vi "Ascenseur_Controller.vi"() -> ()   [LabVIEW 2019]
uses:
  <vilib>/myRIO/Instrument Drivers/Onboard IO/DIO/DIO.lvlib
  Commande 2.ctl
  <vilib>/myRIO/Common/Instrument Driver Framework/myRIO v1.0/DIO/typedefs/DIO Channels Enum.ctl
  <vilib>/myRIO/Common/Instrument Driver Framework/myRIO v1.0/DIO/typedefs/DIO Channels List.ctl
  <vilib>/myRIO/Common/Instrument Driver Framework/Utilities/typedefs/Generic FPGA Reference.ctl
  <vilib>/myRIO/Common/Instrument Driver Framework/Utilities/typedefs/myRIO v1.0 Reference.ctl
  <vilib>/myRIO/Common/Instrument Driver Framework/Utilities/typedefs/Hardware Version Enum.ctl
  <vilib>/myRIO/Common/Instrument Driver Framework/Utilities/typedefs/myRIO Generic Hardware Reference.ctl
  <vilib>/myRIO/Instrument Drivers/Onboard IO/DIO/typedefs/DIO Reference.ctl
  <vilib>/myRIO/Instrument Drivers/Onboard IO/DIO/vis/myRIO DIO Open.xnode
  <vilib>/myRIO/Common/Instrument Driver Framework/myRIO v1.0/DIO/vis/myRIO v1.1 Open DIO.vi
  <vilib>/userDefined/High Color/nirio_resource_hc.ctl
  L298N_Driver/L298N_Ref_Type.ctl
panel:
  in  "Bouton Stop":bool
  out "Var_Etat":T1
  in  "PF_0":bool
  in  "PF_3":bool
  in  "PF_2":bool
  in  "PF_1":bool
  in  "PO_0":bool
  in  "PO_3":bool
  in  "PO_2":bool
  in  "PO_1":bool
  out "Moteur Porte 3":bool
  out "Moteur Porte 2":bool
  out "Moteur Porte 1":bool
  out "Moteur Porte 0":bool
  out "Moteur Cabine":bool
  in  "P0":bool
  in  "P3":bool
  in  "P2":bool
  in  "P1":bool
  in  "Etat_Asc":T1
  in  "Dest_3":bool
  in  "Dest_2":bool
  in  "Dest_1":bool
  in  "Dest_0":bool
  in  "Appel_0":bool
  in  "Appel_3":bool
  in  "Appel_2":bool
  in  "Appel_1":bool
  out "Cluster":T2
  in  "Énum":T3(ring)
  out "Etat":string
  out "Etat Ouvrir Porte 1":bool
  in  "Ouvrir Porte 1":bool
  out "error out 4":errorcluster caption="error out"
  in  "error in (no error) 4":errorcluster caption="error in (no error)"
  in  "Fermer  Porte 1":bool
  out "error out 3":errorcluster caption="error out"
  in  "error in (no error) 3":errorcluster caption="error in (no error)"
  out "error out 2":errorcluster caption="error out"
  in  "error in (no error) 2":errorcluster caption="error in (no error)"
  in  "Cabine Descendre":bool
  out "error out":errorcluster
  in  "error in (no error)":errorcluster
  in  "Cabine Monter":bool
  # "Simulation de présence cabine"
  # "Simulation de portes"
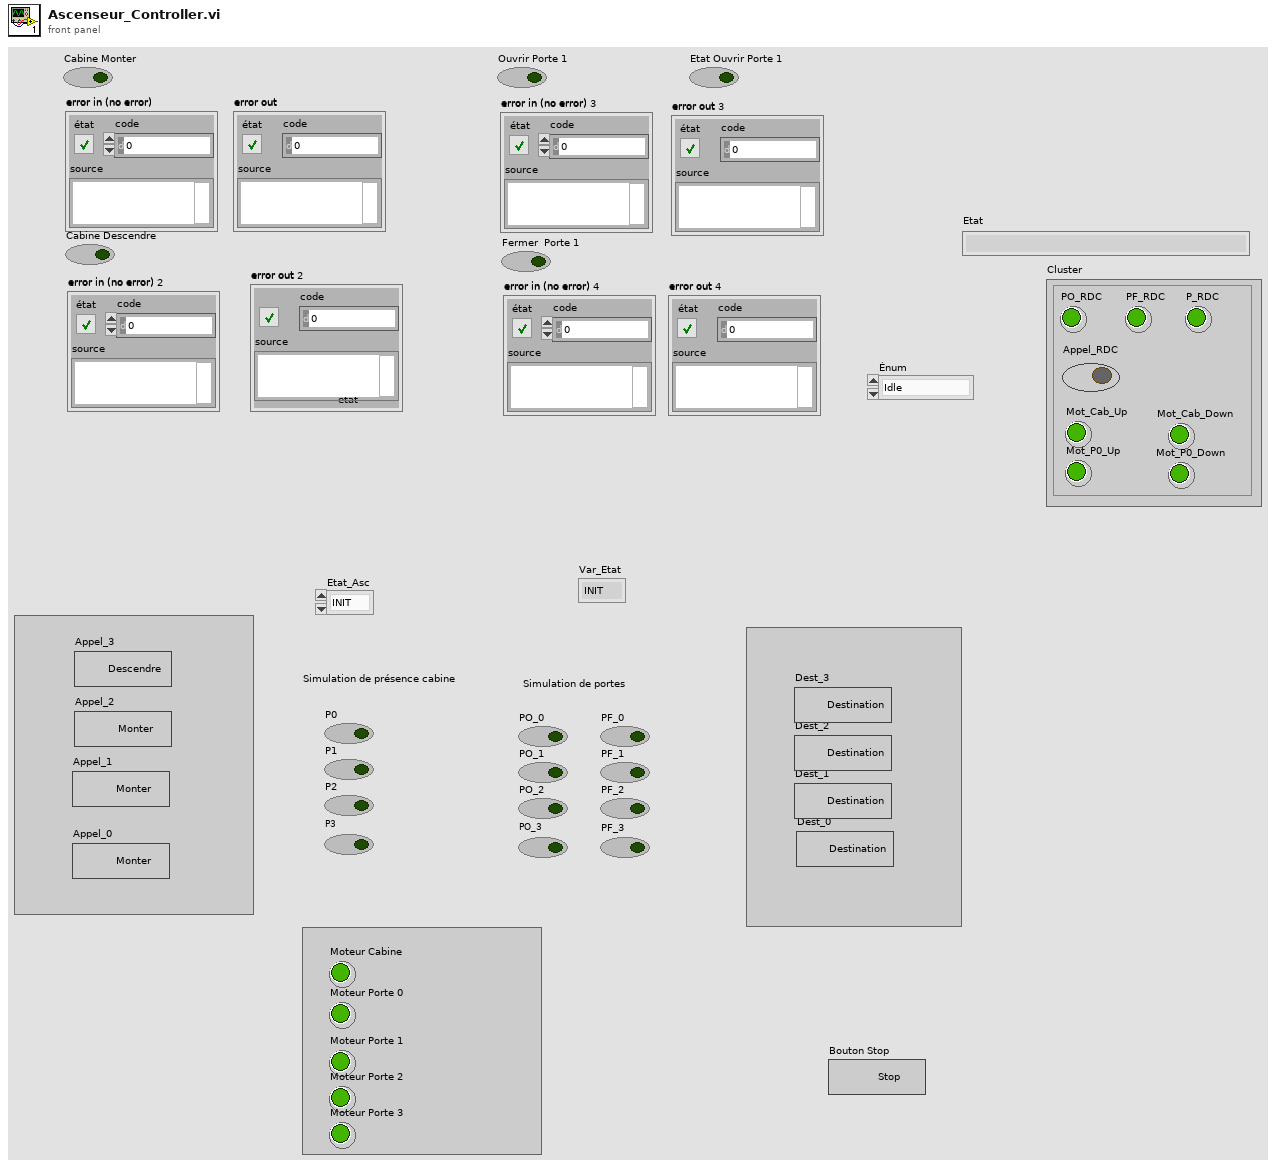
[diagram p1: front panel]
types:
  T1 = typedef "Commande 2.ctl" = enum16{"INIT", "REPOS", "DEPLACEMENT", "OUVERTURE_PORTE", "ATTENTE_TEMPO", "FERMETURE_PORTE", "ARRET_URGENCE"}
  T2 = cluster{"PO_RDC":bool, "PF_RDC":bool, "P_RDC":bool, "Appel_RDC":bool, "Mot_Cab_Up":bool, "Mot_Cab_Down":bool, "Mot_P0_Up":bool, "Mot_P0_Down":bool}
  T3 = enum16{"Idle", "Appel_Etage0", "Descente_Cabine", "Arrivee_Etage0", "Ouverture_Porte", "Attente_Porte", "Fermerture_Porte", "Fin", ""}
  T4 = typedef "L298N_Ref_Type.ctl" = cluster{"DIO_Ref_Montee":T5, "DIO_Ref_Descente":T5}
  T5 = typedef "DIO.lvlib/DIO Reference.ctl" = cluster{"myRIO Reference":T6, "DIO Channels List":T10}
  T6 = typedef "myRIO Generic Hardware Reference.ctl" = cluster{"myRIO Model":T7, "myRIO Hardware Reference":T8}
  T7 = typedef "Hardware Version Enum.ctl" = enum16{"Unknown", "myRIO-1900", "myRIO-1950", "roboRIO", "NI ELVIS RIO CM", "ELVIS III"}
  T8 = typedef "myRIO v1.0 Reference.ctl" = cluster{"Generic FPGA Reference":T9, "Allow multiple opens":bool}
  T9 = typedef "Generic FPGA Reference.ctl" = refnum<k20>
  T10 = typedef "DIO Channels List.ctl" = T11[]
  T11 = typedef "DIO Channels Enum.ctl" = enum16{"Not Connected", "C/DIO0", "C/DIO1", "C/DIO2", "C/DIO3", "C/DIO4", "C/DIO5", "C/DIO6", "C/DIO7", "A/DIO0", "A/DIO1", "A/DIO2", "A/DIO3", "A/DIO4", "A/DIO5", "A/DIO6", "A/DIO7", "A/DIO8", "A/DIO9", "A/DIO10", "A/DIO11", "A/DIO12", "A/DIO13", "A/DIO14", "A/DIO15", "A/DIO16", "A/DIO17", "A/DIO18", "A/DIO19", "B/DIO0", "B/DIO1", "B/DIO2", "B/DIO3", "B/DIO4", "B/DIO5", "B/DIO6", "B/DIO7", "B/DIO8", "B/DIO9", "B/DIO10", "B/DIO11", "B/DIO12", "B/DIO13", "B/DIO14", "B/DIO15", "B/DIO16", "B/DIO17", "B/DIO18", "B/DIO19", "LED0", "LED1", "LED2", "LED3", "Button0", "DIO/DIO0", "DIO/DIO1", "DIO/DIO2", "DIO/DIO3", "DIO/DIO4", "DIO/DIO5", "DIO/DIO6", "DIO/DIO7", "DIO/DIO8", "DIO/DIO9", "SPI/CS0", "SPI/CS1", "SPI/CS2", "SPI/CS3", "LED RADIO (Green)", "LED RADIO (Red)", "LED COMM (Green)", "LED COMM (Red)", "LED MODE (Green)", "LED MODE (Red)"}
  T12 = typedef "nirio_resource_hc.ctl" = tag
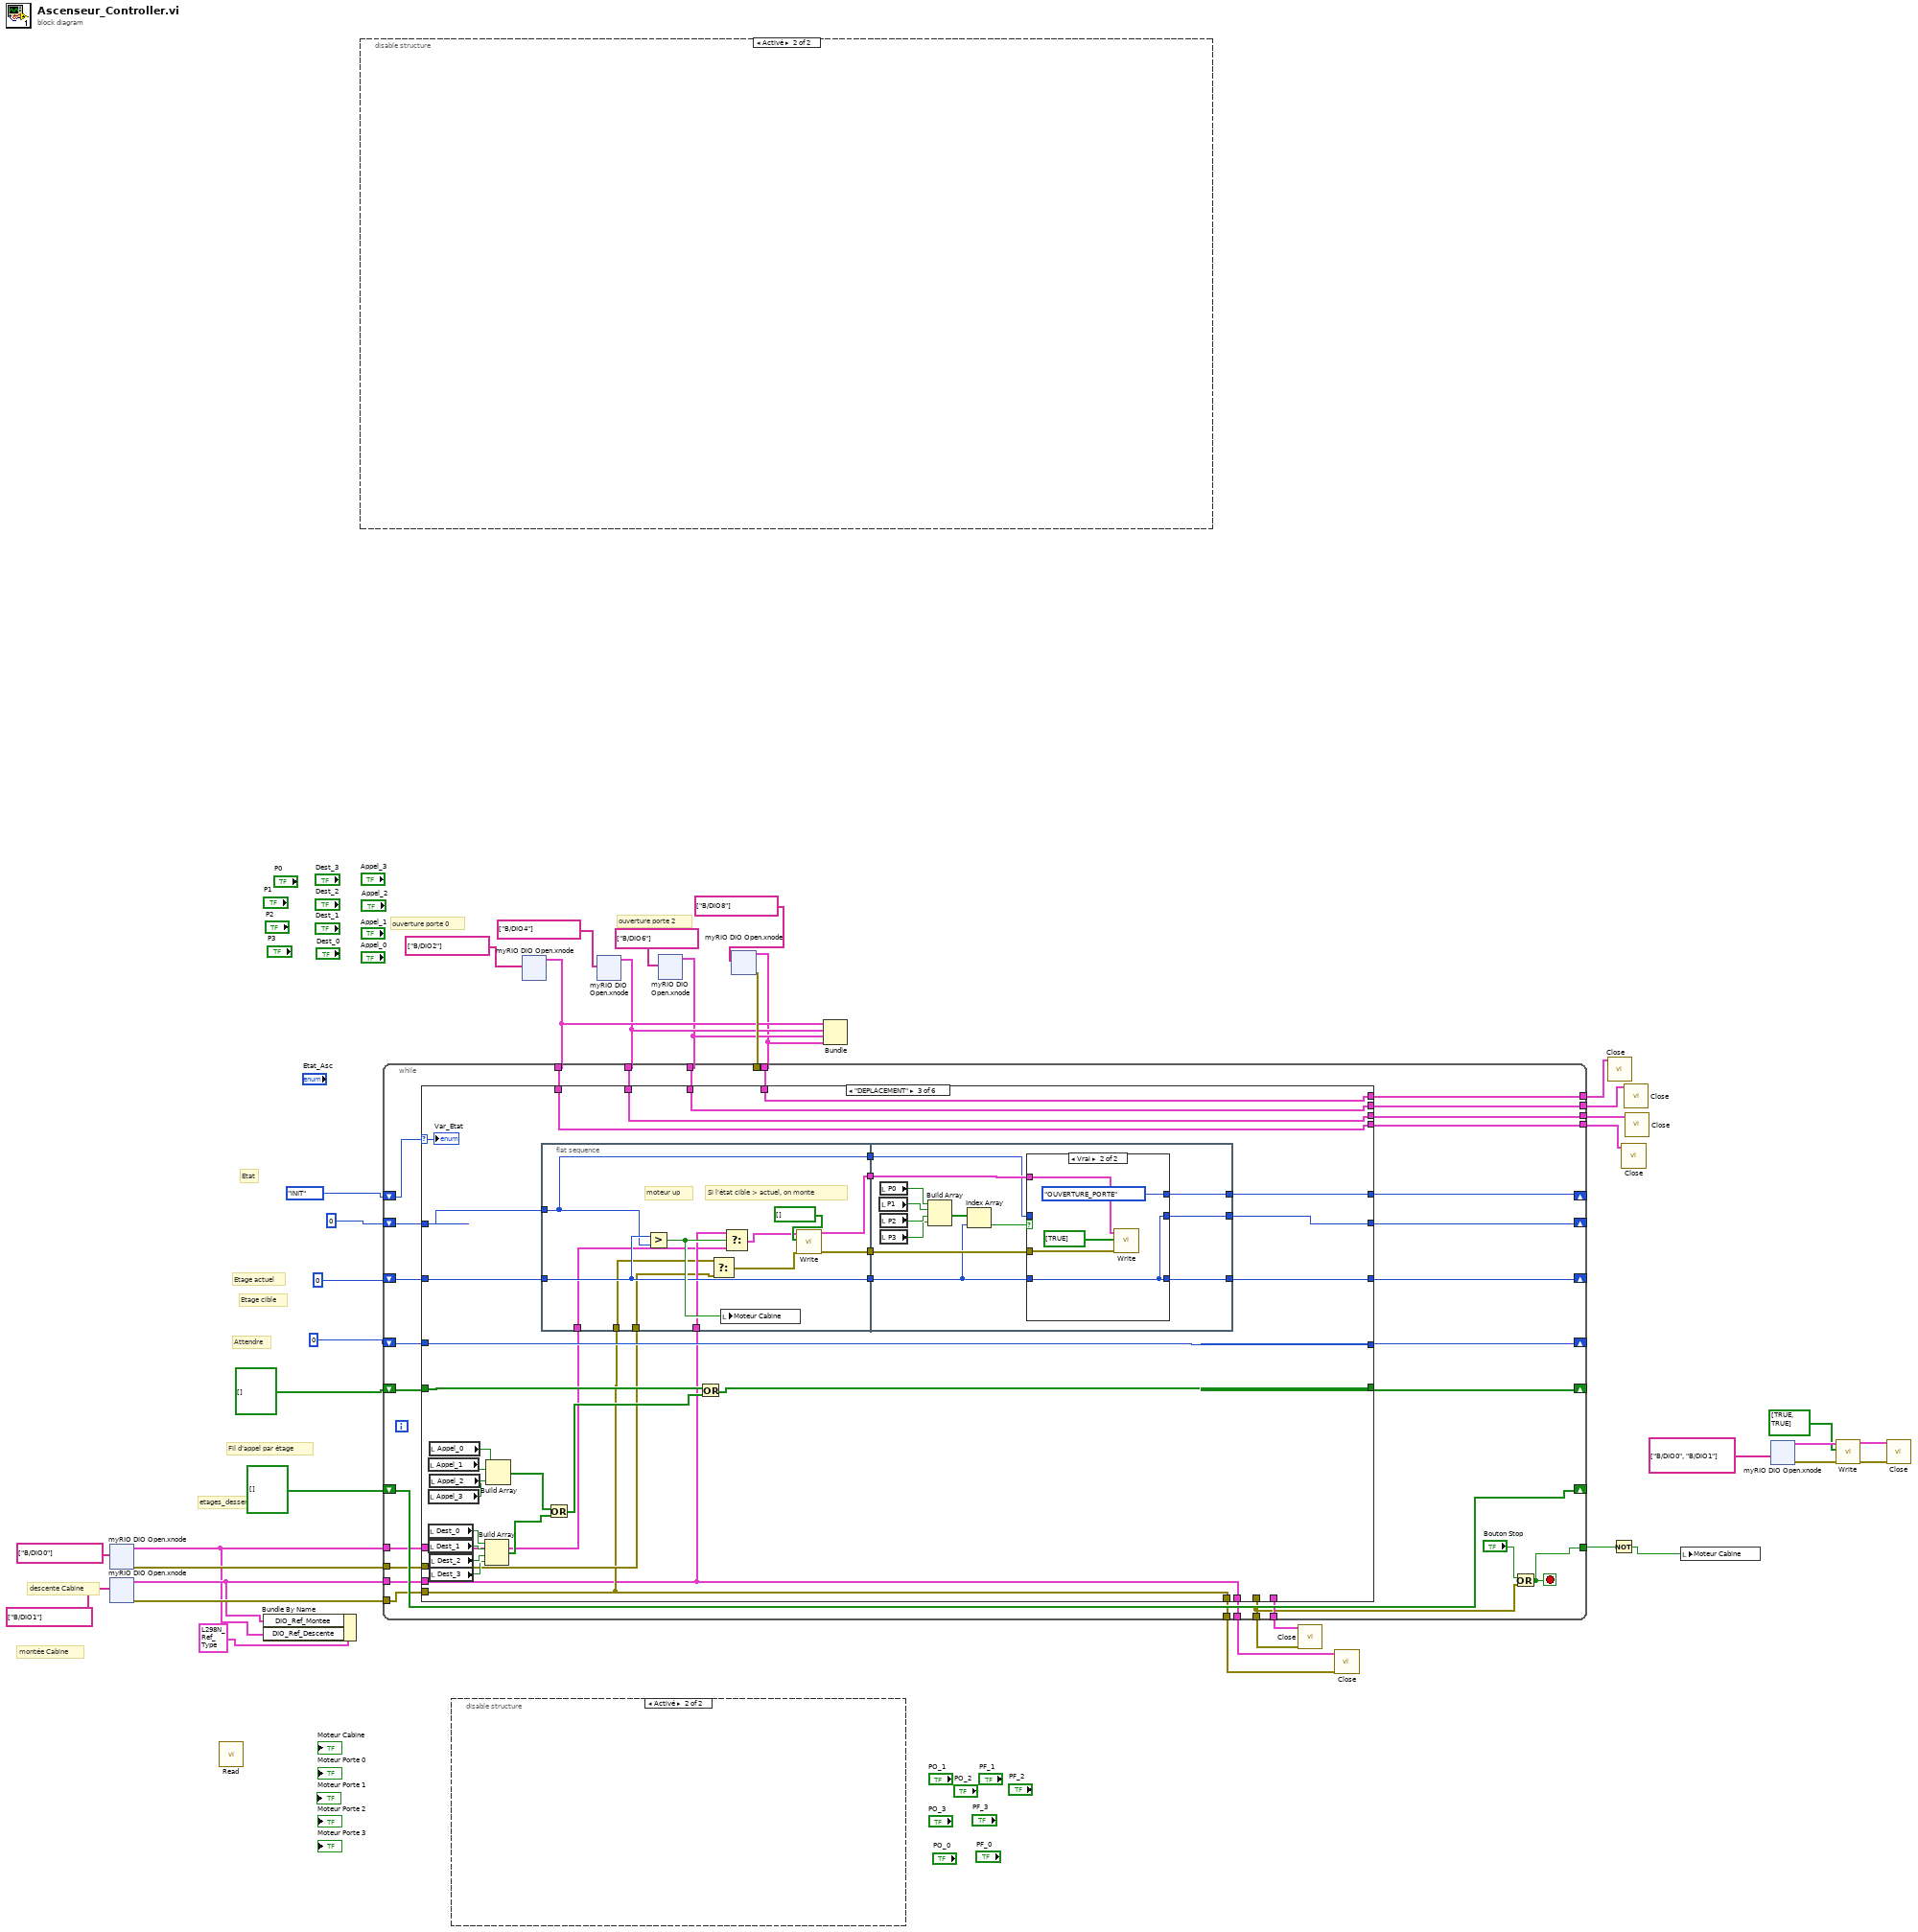
[diagram p0: block diagram]
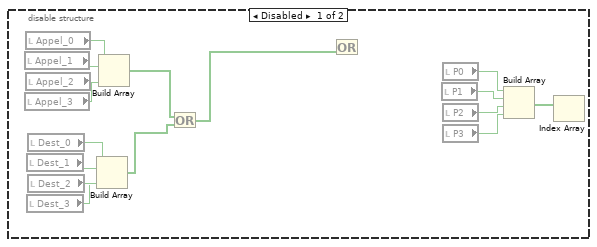
[diagram p2: hidden frame]
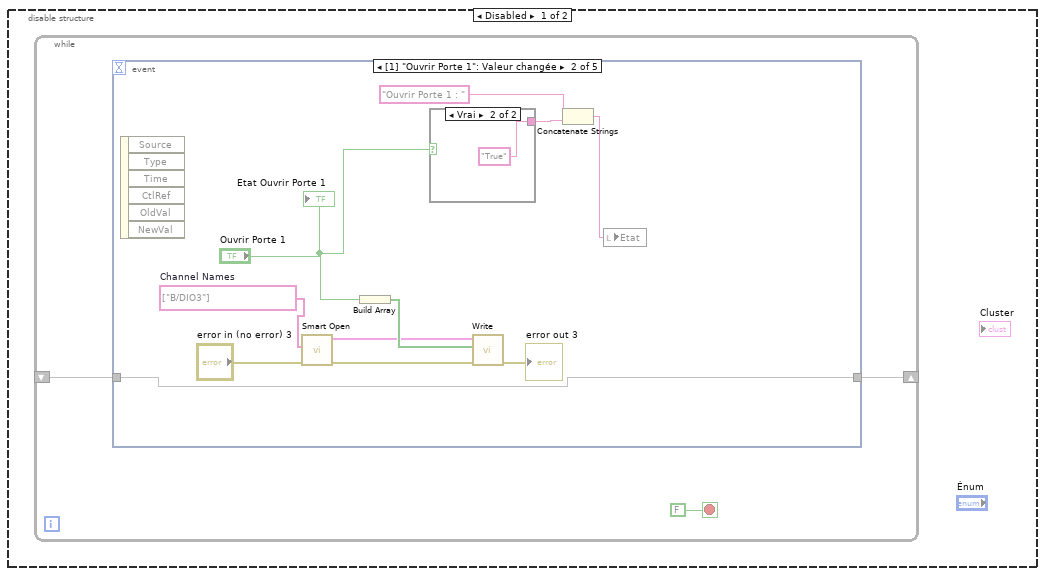
[diagram p3: hidden frame]
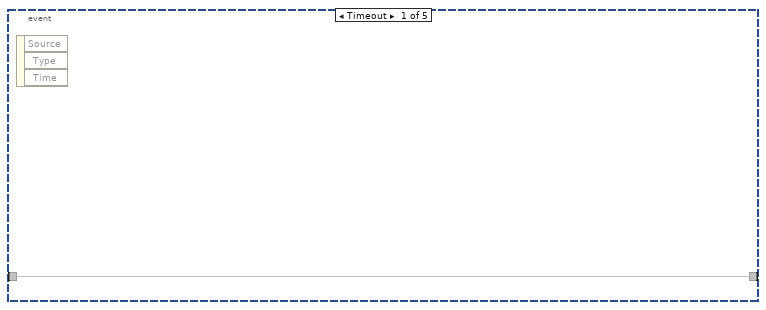
[diagram p4: hidden frame]
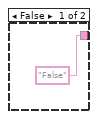
[diagram p5: hidden frame]
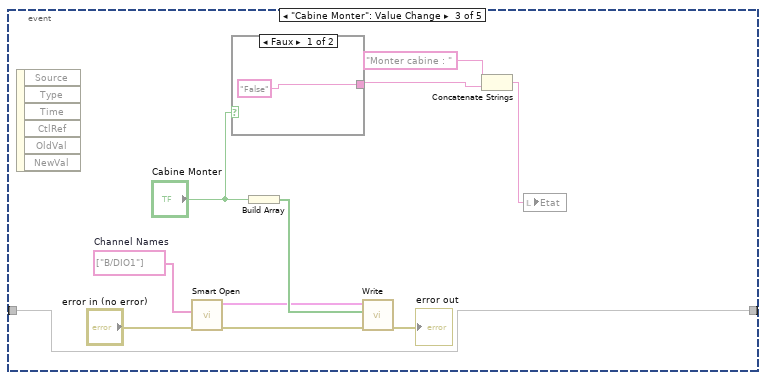
[diagram p6: hidden frame]
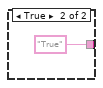
[diagram p7: hidden frame]
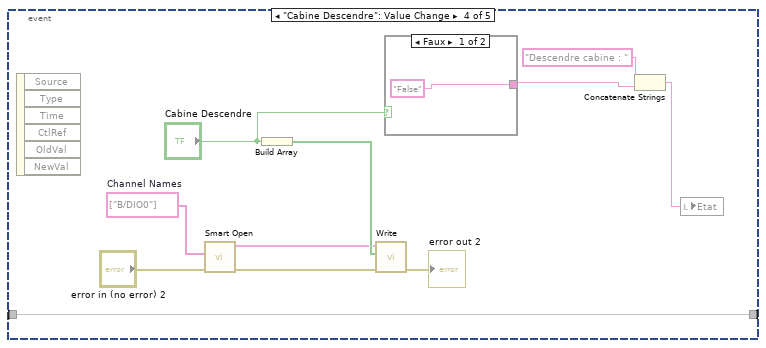
[diagram p8: hidden frame]
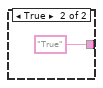
[diagram p9: hidden frame]
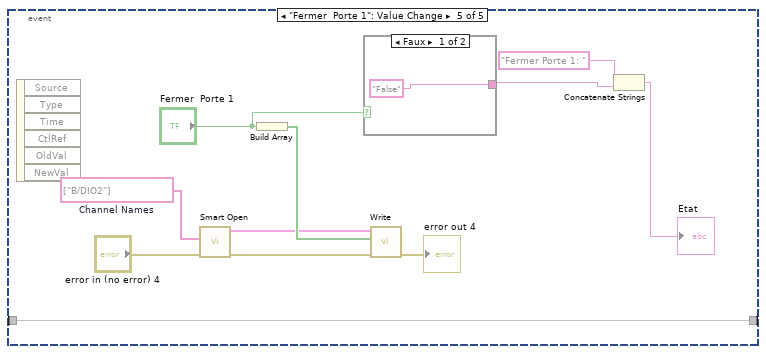
[diagram p10: hidden frame]
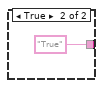
[diagram p11: hidden frame]
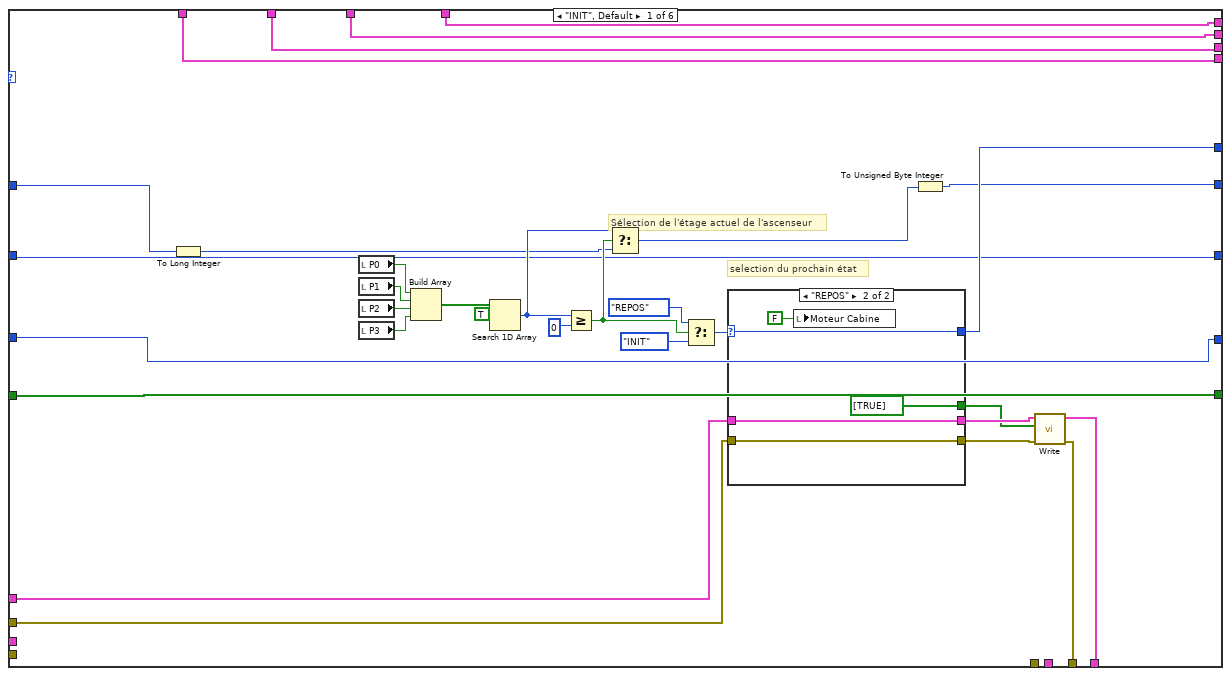
[diagram p12: hidden frame]
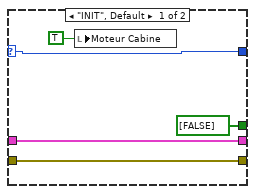
[diagram p13: hidden frame]
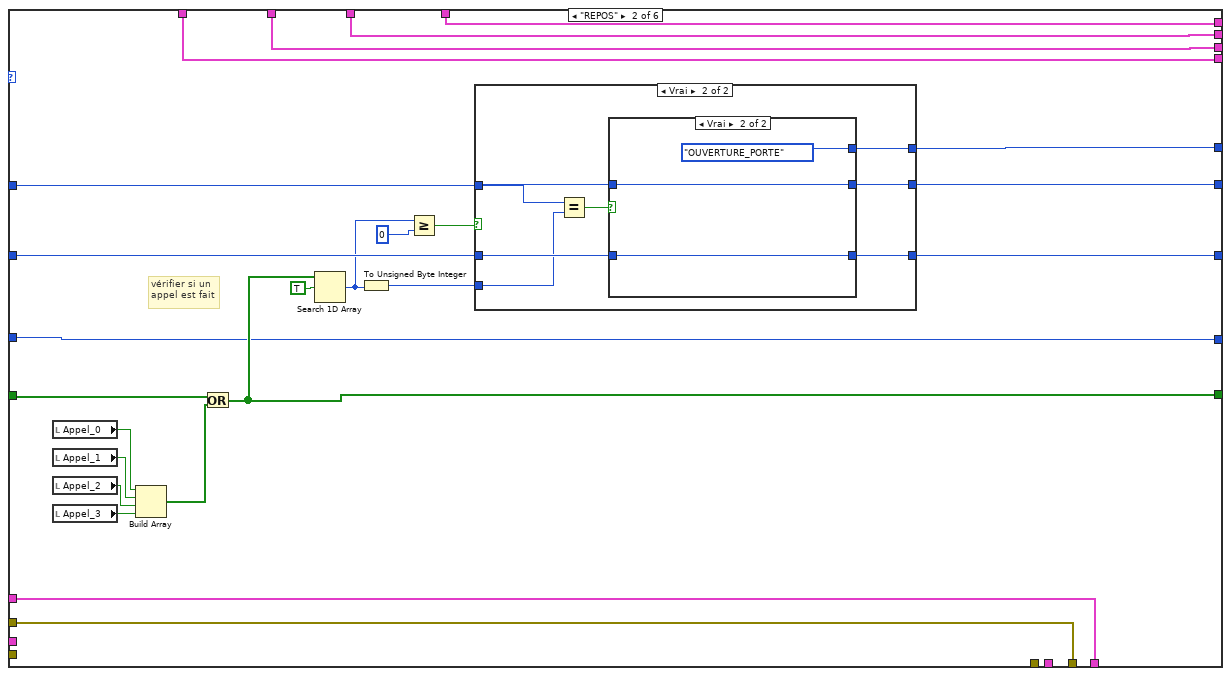
[diagram p14: hidden frame]
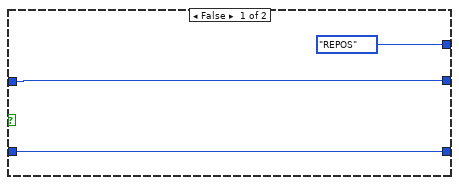
[diagram p15: hidden frame]
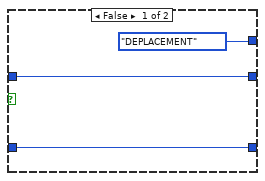
[diagram p16: hidden frame]
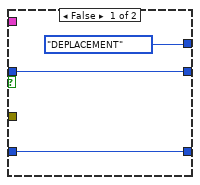
[diagram p17: hidden frame]
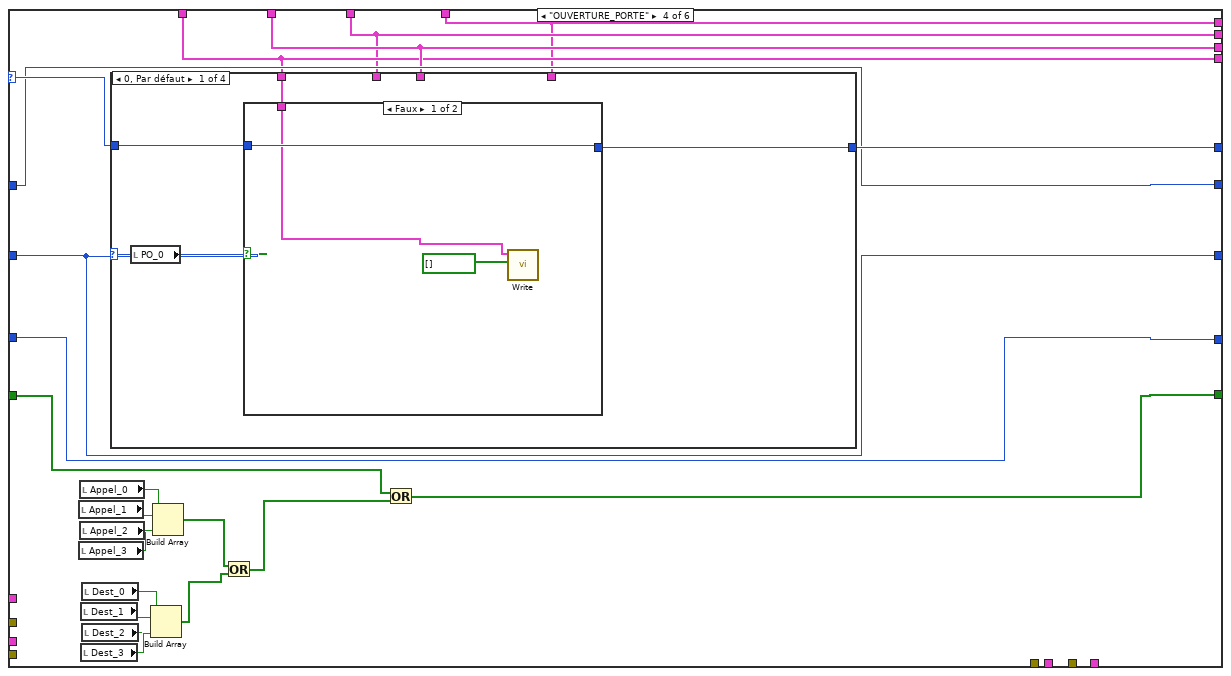
[diagram p18: hidden frame]
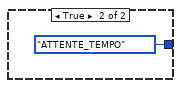
[diagram p19: hidden frame]
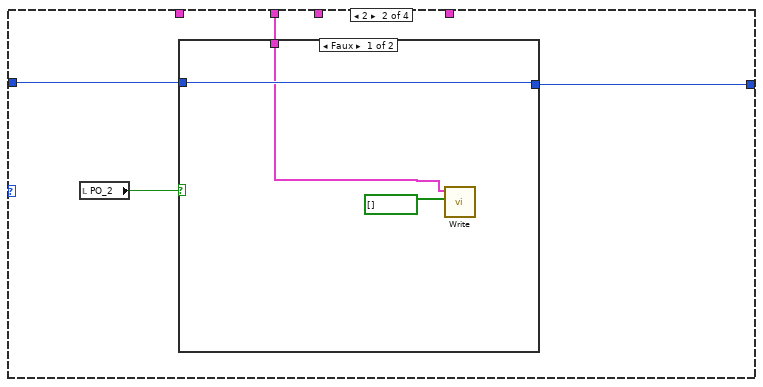
[diagram p20: hidden frame]
diagram:
  # "ouverture porte 2"
  # "ouverture porte 0"
  # "montée Cabine"
  # "descente Cabine"
  # "etages_dessertes"
  # "Fil d'appel par étage"
  # "Attendre"
  # "Etage cible"
  # "Etage actuel"
  # "Etat"
  n1 = xnode "myRIO DIO Open.xnode"("Channel Names"=tag[] ["B/DIO0"]) -> ("error out"=w23:errorcluster, "DIO Ref Out"=w2:T5)  [unwired: 2 in]
  n2 = xnode "myRIO DIO Open.xnode"("Channel Names"=tag[] ["B/DIO1"]) -> ("error out"=w19:errorcluster, "DIO Ref Out"=w3:T5)  [unwired: 2 in]
  n3 = call <vilib>:"Read.vi"() -> ()  [unwired: 9 in, 3 out]
  n4 = Bundle By Name(cluster=T4 {"DIO_Ref_Montee"={"myRIO Reference"={"myRIO Model"=enum."Unknown", "myRIO Hardware Reference"={"Generic FPGA Reference"=refnum, "Allow multiple opens"=FALSE}}, "DIO Channels List"=[]}, "DIO_Ref_Descente"={"myRIO Reference"={"myRIO Model"=enum."Unknown", "myRIO Hardware Reference"={"Generic FPGA Reference"=refnum, "Allow multiple opens"=FALSE}}, "DIO Channels List"=[]}} ("Cluster 2"), "DIO_Ref_Montee"=w3, "DIO_Ref_Descente"=w2) -> ()  [unwired: 1 out]
  n5 = disable-structure shown="Activé" {
    frame Disabled {
      n6 = while {
        shift-right: [w39] -> _
        shift-left: _ -> [w40]
        stop <- FALSE stop-if-true
        n7 = event shown="[1] \"Ouvrir Porte 1\": Valeur changée" {
          selector: _ -> [_ _ _ _ _]
          dyn-events: _ -> [_ _ _ _ _]
          timeout: _ -> [_ _ _ _ _]
          tunnel: [w42 w43 w56 w69 w82] -> w39
          tunnel: w40 -> [w42 w43 w56 w69 w82]
          event Timeout {
            n8 = event-data() -> ()  [unwired: 1 in, 3 out]
          }
          event "Ouvrir Porte 1": Value Change {
            w49 = tag[] ["B/DIO3"]  # Channel Names
            n9 = event-data() -> ()  [unwired: 1 in, 6 out]
            n10 = call <vilib>:"Smart Open.vi"("error in (no error)"="error in (no error) 3", "Channel Names"=w49) -> ("error out"=w50:errorcluster, "DIO Ref Out"=w51:T5)  [unwired: 8 in]
            n11 = Build Array("Ouvrir Porte 1") -> (w53:bool[])
            n12 = case shown="Vrai" "Ouvrir Porte 1" {
              tunnel: ["False" "True"] -> w45
              frame False {
              }
              frame True {
              }
            }
            n13 = call <vilib>:"Write.vi"("error in (no error)"=w50, "Values"=w53, "DIO Ref In"=w51) -> ("error out"=→"error out 3":errorcluster)  [unwired: 6 in, 1 out]
            n14 = Concatenate Strings("Ouvrir Porte 1 : " ("chaîne"), w45) -> (w44:string)
            n15 = local write "Etat"(w44) -> ()
            "Etat Ouvrir Porte 1" <- "Ouvrir Porte 1"
          }
          event "Cabine Monter": Value Change {
            w61 = tag[] ["B/DIO1"]  # Channel Names
            n16 = event-data() -> ()  [unwired: 1 in, 6 out]
            n17 = call <vilib>:"Smart Open.vi"("error in (no error)"="error in (no error)", "Channel Names"=w61) -> ("error out"=w63:errorcluster, "DIO Ref Out"=w64:T5)  [unwired: 8 in]
            n18 = case shown="Faux" "Cabine Monter" {
              tunnel: ["False" "True"] -> w59
              frame False {
              }
              frame True {
              }
            }
            n19 = Build Array("Cabine Monter") -> (w66:bool[])
            n20 = call <vilib>:"Write.vi"("error in (no error)"=w63, "Values"=w66, "DIO Ref In"=w64) -> ("error out"=→"error out":errorcluster)  [unwired: 6 in, 1 out]
            n21 = Concatenate Strings("Monter cabine : " ("chaîne"), w59) -> (w58:string)
            n22 = local write "Etat"(w58) -> ()
          }
          event "Cabine Descendre": Value Change {
            w74 = tag[] ["B/DIO0"]  # Channel Names
            n23 = event-data() -> ()  [unwired: 1 in, 6 out]
            n24 = call <vilib>:"Smart Open.vi"("error in (no error)"="error in (no error) 2", "Channel Names"=w74) -> ("error out"=w76:errorcluster, "DIO Ref Out"=w77:T5)  [unwired: 8 in]
            n25 = Build Array("Cabine Descendre") -> (w79:bool[])
            n26 = call <vilib>:"Write.vi"("error in (no error)"=w76, "Values"=w79, "DIO Ref In"=w77) -> ("error out"=→"error out 2":errorcluster)  [unwired: 6 in, 1 out]
            n27 = case shown="Faux" "Cabine Descendre" {
              tunnel: ["False" "True"] -> w72
              frame False {
              }
              frame True {
              }
            }
            n28 = Concatenate Strings("Descendre cabine : " ("chaîne"), w72) -> (w71:string)
            n29 = local write "Etat"(w71) -> ()
          }
          event "Fermer  Porte 1": Value Change {
            w87 = tag[] ["B/DIO2"]  # Channel Names
            n30 = event-data() -> ()  [unwired: 1 in, 6 out]
            n31 = call <vilib>:"Smart Open.vi"("error in (no error)"="error in (no error) 4", "Channel Names"=w87) -> ("error out"=w89:errorcluster, "DIO Ref Out"=w90:T5)  [unwired: 8 in]
            n32 = Build Array("Fermer  Porte 1") -> (w92:bool[])
            n33 = case shown="Faux" "Fermer  Porte 1" {
              tunnel: ["False" "True"] -> w85
              frame False {
              }
              frame True {
              }
            }
            n34 = call <vilib>:"Write.vi"("error in (no error)"=w89, "Values"=w92, "DIO Ref In"=w90) -> ("error out"=→"error out 4":errorcluster)  [unwired: 6 in, 1 out]
            n35 = Concatenate Strings("Fermer Porte 1: " ("chaîne"), w85) -> (→"Etat":string)
          }
        }
      }
    }
    frame Enabled {
    }
  }
  n36 = disable-structure shown="Activé" {
    frame Disabled {
      n37 = local read "Appel_1"() -> (w96:bool)
      n38 = local read "Appel_3"() -> (w98:bool)
      n39 = local read "Appel_0"() -> (w95:bool)
      n40 = local read "Appel_2"() -> (w97:bool)
      n41 = local read "Dest_1"() -> (w101:bool)
      n42 = local read "Dest_3"() -> (w99:bool)
      n43 = local read "Dest_0"() -> (w102:bool)
      n44 = local read "Dest_2"() -> (w100:bool)
      n45 = Build Array(w102, w101, w100, w99) -> (w104:bool[])
      n46 = Build Array(w95, w96, w97, w98) -> (w103:bool[])
      n47 = Or(x=w103, y=w104) -> (x .or. y?=w105:bool[])
      n48 = Or(y=w105) -> ()  [unwired: 1 in, 1 out]
      n49 = local read "P1"() -> (w107:bool)
      n50 = local read "P0"() -> (w106:bool)
      n51 = local read "P2"() -> (w108:bool)
      n52 = local read "P3"() -> (w109:bool)
      n53 = Build Array(w106, w107, w108, w109) -> (w110:bool[])
      n54 = Index Array(array=w110) -> ()  [unwired: 1 in, 1 out]
    }
    frame Enabled {
    }
  }
  n55 = xnode "myRIO DIO Open.xnode"("Channel Names"=tag[] ["B/DIO2"]) -> ("DIO Ref Out"=w7:T5)  [unwired: 2 in, 1 out]
  n56 = xnode "myRIO DIO Open.xnode"("Channel Names"=tag[] ["B/DIO4"]) -> ("DIO Ref Out"=w6:T5)  [unwired: 2 in, 1 out]
  n57 = xnode "myRIO DIO Open.xnode"("Channel Names"=tag[] ["B/DIO6"]) -> ("DIO Ref Out"=w5:T5)  [unwired: 2 in, 1 out]
  n58 = xnode "myRIO DIO Open.xnode"("Channel Names"=tag[] ["B/DIO8"]) -> ("error out"=w12:errorcluster, "DIO Ref Out"=w4:T5)  [unwired: 2 in]
  n59 = while {
    shift-right: [w132] -> _
    shift-left: Commande_2."INIT" ("Etat_Asc") -> [w139]
    shift-right: [w133] -> _
    shift-left: u8 0 -> [w138]
    shift-right: [w134] -> _
    shift-left: u8 0 -> [w137]
    shift-right: [w130] -> _
    shift-left: 0 -> [w136]
    shift-right: [w131] -> _
    shift-left: bool[] [] -> [w135]
    shift-right: [w129] -> _
    shift-left: bool[] [] -> [w129]
    tunnel: [w126] -> w26
    tunnel: w2 -> [w123]
    tunnel: w23 -> [w124]
    tunnel: [w125] -> w22
    tunnel: [w128] -> w21
    tunnel: w3 -> [w122]
    tunnel: w19 -> [w121]
    tunnel: [w120] -> w18
    tunnel: [w119] -> w17
    tunnel: w7 -> [w115]
    tunnel: w6 -> [w116]
    tunnel: w5 -> [w117]
    tunnel: w4 -> [w118]
    tunnel: w12 -> [_]
    tunnel: [w114] -> w11
    tunnel: [w113] -> w10
    tunnel: [w112] -> w9
    tunnel: [w111] -> w8
    stop <- w126 stop-if-true
    n60 = case shown="\"DEPLACEMENT\"" w139 {
      selector: w139 -> [_ _ w229 w307 _ w368]
      tunnel: w138 -> [w162 w189 w246 w305 w359 w369]
      tunnel: [w160 w200 w236 w306 Commande_2."FERMETURE_PORTE" ("Etat_Asc") w367] -> w132
      tunnel: w137 -> [w159 w198 w247 w304 w358 w366]
      tunnel: [w159 w199 w244 w304 w358 w366] -> w134
      tunnel: w136 -> [w148 w187 w248 w303 w357 w365]
      tunnel: [w158 w195 w237 w290 w343 w370] -> w131
      tunnel: w135 -> [w158 w197 w238 w291 w344 w371]
      tunnel: [w149 w188 w234 w305 w359 w369] -> w133
      tunnel: [w148 w187 w248 w303 w357 w365] -> w130
      tunnel: [w147 w186 _ _ _ _] -> w125
      tunnel: [w146 w185 _ _ _ _] -> w128
      tunnel: w124 -> [w145 w186 w227 _ _ _]
      tunnel: w123 -> [w144 w185 w228 _ _ _]
      tunnel: w122 -> [_ _ w225 _ _ _]
      tunnel: w121 -> [_ _ w226 _ _ _]
      tunnel: [_ _ w225 _ _ _] -> w120
      tunnel: [_ _ w226 _ _ _] -> w119
      tunnel: [w143 w184 w224 w286 w339 w364] -> w114
      tunnel: w118 -> [w143 w184 w224 w286 w339 w364]
      tunnel: [w142 w183 w223 w287 w340 w363] -> w113
      tunnel: w117 -> [w142 w183 w223 w287 w340 w363]
      tunnel: [w141 w182 w222 w289 w341 w362] -> w112
      tunnel: w116 -> [w141 w182 w222 w289 w341 w362]
      tunnel: [w140 w181 w221 w288 w342 w361] -> w111
      tunnel: w115 -> [w140 w181 w221 w288 w342 w361]
      frame "INIT", Default {
        # "Sélection de l'étage actuel de l'ascenseur"
        # "selection du prochain état"
        n61 = To Long Integer(number=w162) -> (32bit integer=w163:i32)
        n62 = local read "P0"() -> (w157:bool)
        n63 = local read "P1"() -> (w156:bool)
        n64 = local read "P2"() -> (w155:bool)
        n65 = local read "P3"() -> (w154:bool)
        n66 = Build Array(w157, w156, w155, w154) -> (w170:bool[])
        n67 = Search 1D Array(1D array=w170, element=TRUE ("élément")) -> (index of element=w164:i32)  [unwired: 1 in]
        n68 = Greater Or Equal?(x=w164, y=0) -> (x >= y?=w165:bool)
        n69 = Select(t=w164, s=w165, f=w163) -> (s? t:f=w150:i32)
        n70 = Select(t=Commande_2."REPOS" ("Etat_Asc"), s=w165, f=Commande_2."INIT" ("Etat_Asc")) -> (s? t:f=w161:T1)
        n71 = case shown="\"REPOS\"" w161 {
          selector: w161 -> [w174 w180]
          tunnel: [w174 w180] -> w160
          tunnel: w144 -> [w173 w178]
          tunnel: w145 -> [w172 w177]
          tunnel: [w173 w178] -> w153
          tunnel: [w172 w177] -> w152
          tunnel: [bool[] [FALSE] ("Values") bool[] [TRUE] ("Values")] -> w151
          frame "INIT", Default {
            n72 = local write "Moteur Cabine"(TRUE ("Moteur Cabine")) -> ()
          }
          frame "REPOS" {
            n73 = local write "Moteur Cabine"(FALSE ("Moteur Cabine")) -> ()
          }
        }
        n74 = To Unsigned Byte Integer(number=w150) -> (unsigned 8bit integer=w149:u8)
        n75 = call <vilib>:"Write.vi"("error in (no error)"=w152, "Values"=w151, "DIO Ref In"=w153) -> ("error out"=w147:errorcluster, "DIO Ref Out"=w146:T5)  [unwired: 6 in]
      }
      frame "REPOS" {
        # "vérifier si un appel est fait"
        n76 = local read "Appel_0"() -> (w204:bool)
        n77 = local read "Appel_1"() -> (w203:bool)
        n78 = local read "Appel_2"() -> (w202:bool)
        n79 = local read "Appel_3"() -> (w201:bool)
        n80 = Build Array(w204, w203, w202, w201) -> (w196:bool[])
        n81 = Or(x=w197, y=w196) -> (x .or. y?=w195:bool[])
        n82 = Search 1D Array(1D array=w195, element=TRUE ("élément")) -> (index of element=w193:i32)  [unwired: 1 in]
        n83 = To Unsigned Byte Integer(number=w193) -> (unsigned 8bit integer=w190:u8)
        n84 = Greater Or Equal?(x=w193, y=0) -> (x >= y?=w191:bool)
        n85 = case shown="Vrai" w191 {
          tunnel: [Commande_2."REPOS" ("Etat_Asc") w213] -> w200
          tunnel: [w206 w212] -> w199
          tunnel: w198 -> [w206 w211]
          tunnel: w190 -> [_ w210]
          tunnel: w189 -> [w205 w208]
          tunnel: [w205 w209] -> w188
          frame False {
          }
          frame True {
            n86 = Equal?(x=w208, y=w210) -> (x = y?=w214:bool)
            n87 = case shown="Vrai" w214 {
              tunnel: [Commande_2."DEPLACEMENT" ("Etat_Asc") Commande_2."OUVERTURE_PORTE" ("Etat_Asc")] -> w213
              tunnel: [w215 w219] -> w212
              tunnel: w211 -> [w215 w219]
              tunnel: w208 -> [w216 w218]
              tunnel: [w216 w218] -> w209
              frame False {
              }
              frame True {
              }
            }
          }
        }
      }
      frame "DEPLACEMENT" {
        n88 = local read "Appel_1"() -> (w251:bool)
        n89 = local read "Appel_3"() -> (w249:bool)
        n90 = local read "Dest_0"() -> (w233:bool)
        n91 = local read "Dest_1"() -> (w232:bool)
        n92 = local read "Appel_0"() -> (w252:bool)
        n93 = local read "Appel_2"() -> (w250:bool)
        n94 = local read "Dest_2"() -> (w231:bool)
        n95 = local read "Dest_3"() -> (w230:bool)
        n96 = Build Array(w233, w232, w231, w230) -> (w240:bool[])
        n97 = Build Array(w252, w251, w250, w249) -> (w241:bool[])
        n98 = flat-sequence {
          tunnel: w246 -> [w259]
          tunnel: w247 -> [w262]
          tunnel: [w262] -> w245
          tunnel: [w261] -> w243
          tunnel: [w260] -> w242
          tunnel: [w259] -> w235
          tunnel: w225 -> [w257]
          tunnel: w228 -> [w256]
          tunnel: w226 -> [w255]
          tunnel: w227 -> [w254]
          tunnel: w245 -> [w265]
          tunnel: [w266] -> w244
          tunnel: w243 -> [w271]
          tunnel: w242 -> [w270]
          tunnel: [w269] -> w236
          tunnel: w235 -> [w268]
          tunnel: [w267] -> w234
          frame #0 {
            # "Si l'état cible > actuel, on monte"
            # "moteur up"
            n99 = Greater?(x=w262, y=w259) -> (0:w263:bool)
            n100 = Select(t=w255, f=w254) -> (s? t:f=w253:errorcluster)  [unwired: 1 in]
            n101 = local write "Moteur Cabine"(w263) -> ()
            n102 = Select(t=w257, s=w263, f=w256) -> (s? t:f=w258:T5)
            n103 = call <vilib>:"Write.vi"("error in (no error)"=w253, "Values"=bool[] [], "DIO Ref In"=w258) -> ("error out"=w261:errorcluster, "DIO Ref Out"=w260:T5)  [unwired: 6 in]
          }
          frame #1 {
            n104 = local read "P1"() -> (w276:bool)
            n105 = local read "P0"() -> (w277:bool)
            n106 = local read "P2"() -> (w275:bool)
            n107 = local read "P3"() -> (w274:bool)
            n108 = Build Array(w277, w276, w275, w274) -> (w273:bool[])
            n109 = Index Array(array=w273, index=w265) -> (element=w272:bool)
            n110 = case shown="Vrai" w272 {
              tunnel: w271 -> [_ w285]
              tunnel: w270 -> [_ w283]
              tunnel: [Commande_2."DEPLACEMENT" ("Etat_Asc") Commande_2."OUVERTURE_PORTE" ("Etat_Asc")] -> w269
              tunnel: w268 -> [w279 _]
              tunnel: [w279 w281] -> w267
              tunnel: [w278 w281] -> w266
              tunnel: w265 -> [w278 w281]
              frame False {
              }
              frame True {
                n111 = call <vilib>:"Write.vi"("error in (no error)"=w285, "Values"=bool[] [TRUE], "DIO Ref In"=w283) -> ()  [unwired: 6 in, 2 out]
              }
            }
          }
        }
        n112 = Or(x=w241, y=w240) -> (x .or. y?=w239:bool[])
        n113 = Or(x=w238, y=w239) -> (x .or. y?=w237:bool[])
        "Var_Etat" <- w229
      }
      frame "OUVERTURE_PORTE" {
        n114 = local read "Appel_1"() -> (w301:bool)
        n115 = local read "Appel_3"() -> (w299:bool)
        n116 = local read "Appel_0"() -> (w302:bool)
        n117 = local read "Appel_2"() -> (w300:bool)
        n118 = local read "Dest_1"() -> (w296:bool)
        n119 = local read "Dest_3"() -> (w298:bool)
        n120 = local read "Dest_0"() -> (w295:bool)
        n121 = local read "Dest_2"() -> (w297:bool)
        n122 = case shown="0, Par défaut" w304 {
          tunnel: w307 -> [w309 w318 w325 w332]
          tunnel: [w310 w319 w326 w333] -> w306
          tunnel: w289 -> [_ _ _ w331]
          tunnel: w288 -> [w308 _ _ _]
          tunnel: w287 -> [_ w316 _ _]
          tunnel: w286 -> [_ _ w324 _]
          frame 0, Default {
            n123 = local read "PO_0"() -> (w311:bool)
            n124 = case shown="Faux" w311 {
              tunnel: w309 -> [w314 _]
              tunnel: [w314 Commande_2."ATTENTE_TEMPO" ("Etat_Asc")] -> w310
              tunnel: w308 -> [w312 _]
              frame False {
                n125 = call <vilib>:"Write.vi"("Values"=bool[] [], "DIO Ref In"=w312) -> ()  [unwired: 7 in, 2 out]
              }
              frame True {
              }
            }
          }
          frame 2 {
            n126 = local read "PO_2"() -> (w317:bool)
            n127 = case shown="Faux" w317 {
              tunnel: w318 -> [w322 _]
              tunnel: [w322 Commande_2."ATTENTE_TEMPO" ("Etat_Asc")] -> w319
              tunnel: w316 -> [w320 _]
              frame False {
                n128 = call <vilib>:"Write.vi"("Values"=bool[] [], "DIO Ref In"=w320) -> ()  [unwired: 7 in, 2 out]
              }
              frame True {
              }
            }
          }
          frame 3 {
            n129 = local read "PO_3"() -> (w327:bool)
            n130 = case shown="Faux" w327 {
              tunnel: [w329 Commande_2."ATTENTE_TEMPO" ("Etat_Asc")] -> w326
              tunnel: w325 -> [w329 _]
              tunnel: w324 -> [w328 _]
              frame False {
                n131 = call <vilib>:"Write.vi"("DIO Ref In"=w328) -> ()  [unwired: 8 in, 2 out]
              }
              frame True {
              }
            }
          }
          frame 1 {
            n132 = local read "PO_1"() -> (w334:bool)
            n133 = case shown="Faux" w334 {
              tunnel: [w336 Commande_2."ATTENTE_TEMPO" ("Etat_Asc")] -> w333
              tunnel: w332 -> [w336 _]
              tunnel: w331 -> [w335 _]
              frame False {
                n134 = call <vilib>:"Write.vi"("Values"=bool[] [], "DIO Ref In"=w335) -> ()  [unwired: 7 in, 2 out]
              }
              frame True {
              }
            }
          }
        }
        n135 = Build Array(w295, w296, w297, w298) -> (w293:bool[])
        n136 = Build Array(w302, w301, w300, w299) -> (w294:bool[])
        n137 = Or(x=w294, y=w293) -> (x .or. y?=w292:bool[])
        n138 = Or(x=w291, y=w292) -> (x .or. y?=w290:bool[])
      }
      frame "ATTENTE_TEMPO" {
        n139 = local read "Appel_1"() -> (w354:bool)
        n140 = local read "Appel_3"() -> (w352:bool)
        n141 = local read "Appel_0"() -> (w355:bool)
        n142 = local read "Appel_2"() -> (w353:bool)
        n143 = local read "Dest_1"() -> (w349:bool)
        n144 = local read "Dest_3"() -> (w351:bool)
        n145 = local read "Dest_0"() -> (w348:bool)
        n146 = local read "Dest_2"() -> (w350:bool)
        n147 = Build Array(w348, w349, w350, w351) -> (w346:bool[])
        n148 = Build Array(w355, w354, w353, w352) -> (w347:bool[])
        n149 = Or(x=w347, y=w346) -> (x .or. y?=w345:bool[])
        n150 = Or(x=w344, y=w345) -> (x .or. y?=w343:bool[])
        n151 = Wait (ms)(milliseconds to wait=u32 3000 ("attente (ms)")) -> ()  [unwired: 1 out]
      }
      frame "FERMETURE_PORTE" {
        n152 = local read "Appel_1"() -> (w381:bool)
        n153 = local read "Appel_3"() -> (w379:bool)
        n154 = local read "Appel_0"() -> (w382:bool)
        n155 = local read "Appel_2"() -> (w380:bool)
        n156 = Build Array(w382, w381, w380, w379) -> (w374:bool[])
        n157 = case shown="3" w366 {
          tunnel: w368 -> [w383 w411 w437 w464]
          tunnel: [w384 w412 w438 w465] -> w367
          frame 0, Default {
            n158 = local read "PO_0"() -> (w385:bool)
            n159 = case shown="Vrai" w385 {
              tunnel: w383 -> [w392 _]
              tunnel: [w392 Commande_2."REPOS" ("Etat_Asc")] -> w384
              frame False {
                n160 = xnode "myRIO DIO Open.xnode"("Channel Names"=tag[] ["B/DIO3"]) -> ("error out"=w389:errorcluster, "DIO Ref Out"=w388:T5)  [unwired: 2 in]
                n161 = call <vilib>:"Write.vi"("error in (no error)"=w389, "Values"=bool[] [], "DIO Ref In"=w388) -> ("error out"=w390:errorcluster, "DIO Ref Out"=w391:T5)  [unwired: 6 in]
                n162 = call <vilib>:"Close.vi"("error in (no error)"=w390, "DIO Ref In"=w391) -> ()  [unwired: 9 in, 1 out]
              }
              frame True {
              }
            }
          }
          frame 2 {
            n163 = local read "PO_2"() -> (w410:bool)
            n164 = case shown="Vrai" w410 {
              tunnel: w411 -> [w419 _]
              tunnel: [w419 Commande_2."REPOS" ("Etat_Asc")] -> w412
              frame False {
                n165 = xnode "myRIO DIO Open.xnode"("Channel Names"=tag[] ["B/DIO6"]) -> ("error out"=w416:errorcluster, "DIO Ref Out"=w415:T5)  [unwired: 2 in]
                n166 = call <vilib>:"Write.vi"("error in (no error)"=w416, "Values"=bool[] [], "DIO Ref In"=w415) -> ("error out"=w417:errorcluster, "DIO Ref Out"=w418:T5)  [unwired: 6 in]
                n167 = call <vilib>:"Close.vi"("error in (no error)"=w417, "DIO Ref In"=w418) -> ()  [unwired: 9 in, 1 out]
              }
              frame True {
              }
            }
          }
          frame 3 {
            n168 = local read "PO_3"() -> (w439:bool)
            n169 = case shown="Faux" w439 {
              tunnel: [w440 Commande_2."REPOS" ("Etat_Asc")] -> w438
              tunnel: w437 -> [w440 _]
              frame False {
                n170 = xnode "myRIO DIO Open.xnode"("Channel Names"=tag[] ["B/DIO8"]) -> ("error out"=w444:errorcluster, "DIO Ref Out"=w443:T5)  [unwired: 2 in]
                n171 = call <vilib>:"Write.vi"("error in (no error)"=w444, "Values"=bool[] [], "DIO Ref In"=w443) -> ("error out"=w445:errorcluster, "DIO Ref Out"=w446:T5)  [unwired: 6 in]
                n172 = call <vilib>:"Close.vi"("error in (no error)"=w445, "DIO Ref In"=w446) -> ()  [unwired: 9 in, 1 out]
              }
              frame True {
              }
            }
          }
          frame 1 {
            n173 = local read "PO_1"() -> (w466:bool)
            n174 = case shown="Vrai" w466 {
              tunnel: [w467 Commande_2."REPOS" ("Etat_Asc")] -> w465
              tunnel: w464 -> [w467 _]
              frame False {
                n175 = xnode "myRIO DIO Open.xnode"("Channel Names"=tag[] ["B/DIO4"]) -> ("error out"=w471:errorcluster, "DIO Ref Out"=w470:T5)  [unwired: 2 in]
                n176 = call <vilib>:"Write.vi"("error in (no error)"=w471, "Values"=bool[] [], "DIO Ref In"=w470) -> ("error out"=w472:errorcluster, "DIO Ref Out"=w473:T5)  [unwired: 6 in]
                n177 = call <vilib>:"Close.vi"("error in (no error)"=w472, "DIO Ref In"=w473) -> ()  [unwired: 9 in, 1 out]
              }
              frame True {
              }
            }
          }
        }
        n178 = local read "Dest_1"() -> (w376:bool)
        n179 = local read "Dest_3"() -> (w378:bool)
        n180 = local read "Dest_0"() -> (w375:bool)
        n181 = local read "Dest_2"() -> (w377:bool)
        n182 = Build Array(w375, w376, w377, w378) -> (w373:bool[])
        n183 = Or(x=w374, y=w373) -> (x .or. y?=w372:bool[])
        n184 = Or(x=w371, y=w372) -> (x .or. y?=w370:bool[])
      }
    }
    n185 = Or(x="Bouton Stop", y=w125) -> (x .or. y?=w126:bool)
  }
  n186 = Bundle("DIO Ref Out"=w7, "DIO Ref Out"=w6, "DIO Ref Out"=w5, "DIO Ref Out"=w4) -> ()  [unwired: 1 in, 1 out]
  n187 = call <vilib>:"Close.vi"("error in (no error)"=w22, "DIO Ref In"=w21) -> ()  [unwired: 9 in, 1 out]
  n188 = call <vilib>:"Close.vi"("error in (no error)"=w17, "DIO Ref In"=w18) -> ()  [unwired: 9 in, 1 out]
  n189 = call <vilib>:"Close.vi"("DIO Ref In"=w11) -> ()  [unwired: 10 in, 1 out]
  n190 = Not(x=w26) -> (.not. x?=w25:bool)
  n191 = call <vilib>:"Close.vi"("DIO Ref In"=w8) -> ()  [unwired: 10 in, 1 out]
  n192 = call <vilib>:"Close.vi"("DIO Ref In"=w10) -> ()  [unwired: 10 in, 1 out]
  n193 = call <vilib>:"Close.vi"("DIO Ref In"=w9) -> ()  [unwired: 10 in, 1 out]
  n194 = local write "Moteur Cabine"(w25) -> ()
  n195 = xnode "myRIO DIO Open.xnode"("Channel Names"=tag[] ["B/DIO0", "B/DIO1"]) -> ("error out"=w28:errorcluster, "DIO Ref Out"=w31:T5)  [unwired: 2 in]
  n196 = call <vilib>:"Write.vi"("error in (no error)"=w28, "Values"=bool[] [TRUE, TRUE], "DIO Ref In"=w31) -> ("error out"=w29:errorcluster, "DIO Ref Out"=w30:T5)  [unwired: 6 in]
  n197 = call <vilib>:"Close.vi"("error in (no error)"=w29, "DIO Ref In"=w30) -> ()  [unwired: 9 in, 1 out]
